vi "Display Accele Waveform_SubVIs-某型振动实验台测试系统.vi"(7 "WFGraph Refnum":refnum<vi>, 8 "error in":errorcluster, 10 "Color Array":u32[](array[numeric]), 11 "Data":waveform(dbl)[](array[waveform])) -> (0 "error out":errorcluster)   [LabVIEW 2011]
doc: "将索引出的波形显示在波形图中；\n并设置相应波形显示的颜色。"
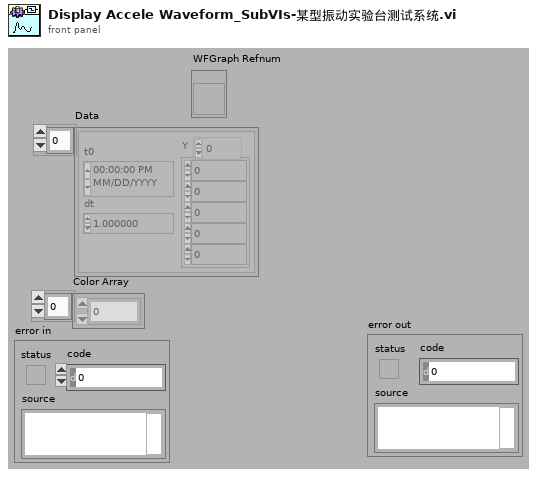
[diagram p1: front panel]
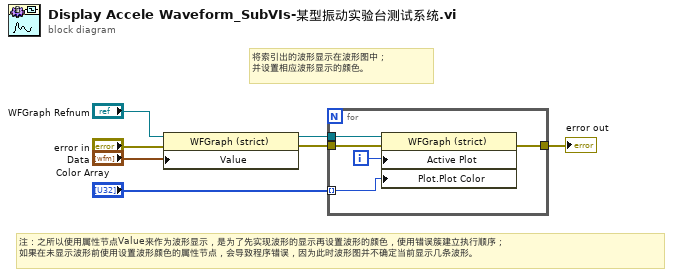
[diagram p0: block diagram]
diagram:
  # "注：之所以使用属性节点Value来作为波形显示，是为了先实现波形的显示再设置波形的颜色，使用错误簇建立执行顺序；\n如果在未显示波形前使用设置波形颜色的属性节点，会导致程序错误，因为此时波形图并不确定当前显示几条波形。"
  # "将索引出的波形显示在波形图中；\n并设置相应波形显示的颜色。"
  n1 = property on="Property Node" class="WFGraph (strict)"(reference="WFGraph Refnum", error in="error in", "Value"="Data") -> (reference out=w1:refnum<vi>, error out=w7:errorcluster)
  n2 = for {
    tunnel: "Color Array" -> [w12] mode=indexing
    tunnel: w7 -> [w10]
    tunnel: w1 -> [w9]
    tunnel: [w8] -> w3
    i -> [w11]
    n3 = property on="Property Node" class="WFGraph (strict)"(reference=w9, error in=w10, "Active Plot"=w11, "Plot.Plot Color"=w12) -> (error out=w8:errorcluster)  [unwired: 1 out]
  }
  "error out" <- w3
